vi "Get Supported Targets.vi"(8 "error in":errorcluster, 11 "System Diagnostics configuration in":refnum<class "System Diagnostics configuration.lvclass">) -> (0 "error out":errorcluster, 2 "supported targets":T1[](array[typedef]), 3 "System Diagnostics configuration out":refnum<class "System Diagnostics configuration.lvclass">)   [LabVIEW 2013, in "System Diagnostics configuration.lvclass"]
doc: "Provides an interface for determining the targets supported by a given module configuration/runtime class pairing. This should be overridden by any useful child class."
uses:
  System Diagnostics configuration.lvclass
  <vilib>/NI/Tag Bus Module Framework/root configuration/Target Types.ctl
  <vilib>/NI/Tag Bus Module Framework/root configuration/TBM configuration.lvclass
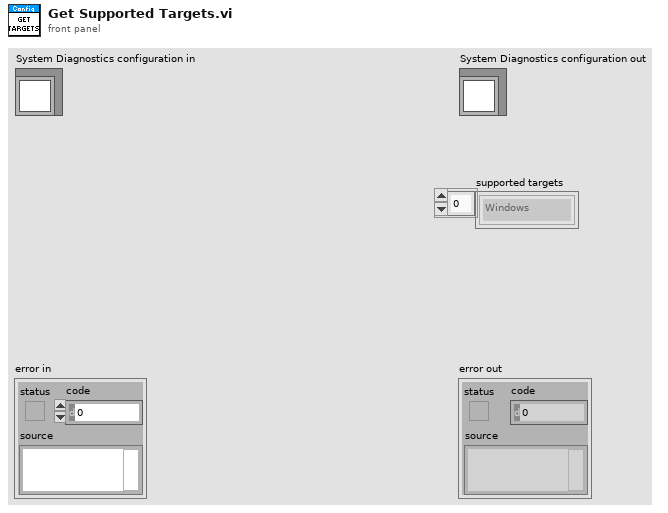
[diagram p1: front panel]
types:
  T1 = typedef "TBM configuration.lvclass/Target Types.ctl" = enum16{"Windows", "Mac", "Linux", "Linux RT ARM", "VxWorks", "Pharlap", "Other", "Linux RT x64"}
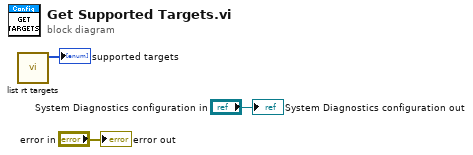
[diagram p0: block diagram]
diagram:
  n1 = call <vilib>:"list rt targets.vi"() -> ("desktop targets"=→"supported targets":T1[])  [unwired: 11 in]
  "error out" <- "error in"
  "System Diagnostics configuration out" <- "System Diagnostics configuration in"
